vi "myRIO_BRig_RT_dataTrial_Cue1_time.vi"() -> (2 "output_Cue1_time":i32)   [LabVIEW 2014]
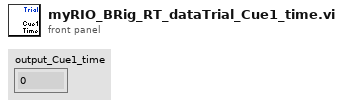
[diagram p1: front panel]
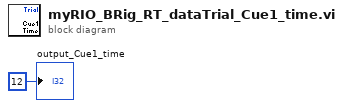
[diagram p0: block diagram]
diagram:
  "output_Cue1_time" <- 12 ("output_iBlock")
